vi "Sub Routing program.vi"(0 "queue Out in":refnum<queue>, 1 "FeedBack Channel":string[](array[string]), 2 "Load":refnum<vi>, 5 "reference in":refnum<vi>, 9 "Feature Step Enable":T1(array[cluster]), 11 "error in (no error)":errorcluster, 12 "Str Refnum":refnum<vi>, 14 "Pict Refnum":refnum<vi>) -> (3 "2D Picture":picture, 4 "Queue out":refnum<queue>, 6 "reference out":refnum<vi>, 10 "Result":bool, 15 "error out":errorcluster)   [LabVIEW 2015]
uses:
  Test  enqueue/AutoTest seq.ctl
  Galobal variable_TI.vi
  Project Setup/Globle Variable/GR_Servo.vi
panel:
  out "error out 2":errorcluster
  in  "Select Part":u16(ring) items=["CHECK BARCODE.jpg", "Difusser.jpg", "FIX BLACK PART.jpg", "FIXED PCB.jpg", "INSER KEYPAD.jpg", "IONIZE PCB.jpg", "light box ionization.jpg", "MOVE DOWN PART.jpg", "MOVING PART.jpg", "PART.jpg", "PUT PART ON FIXTURE.jpg"]
  out "Error Message":string
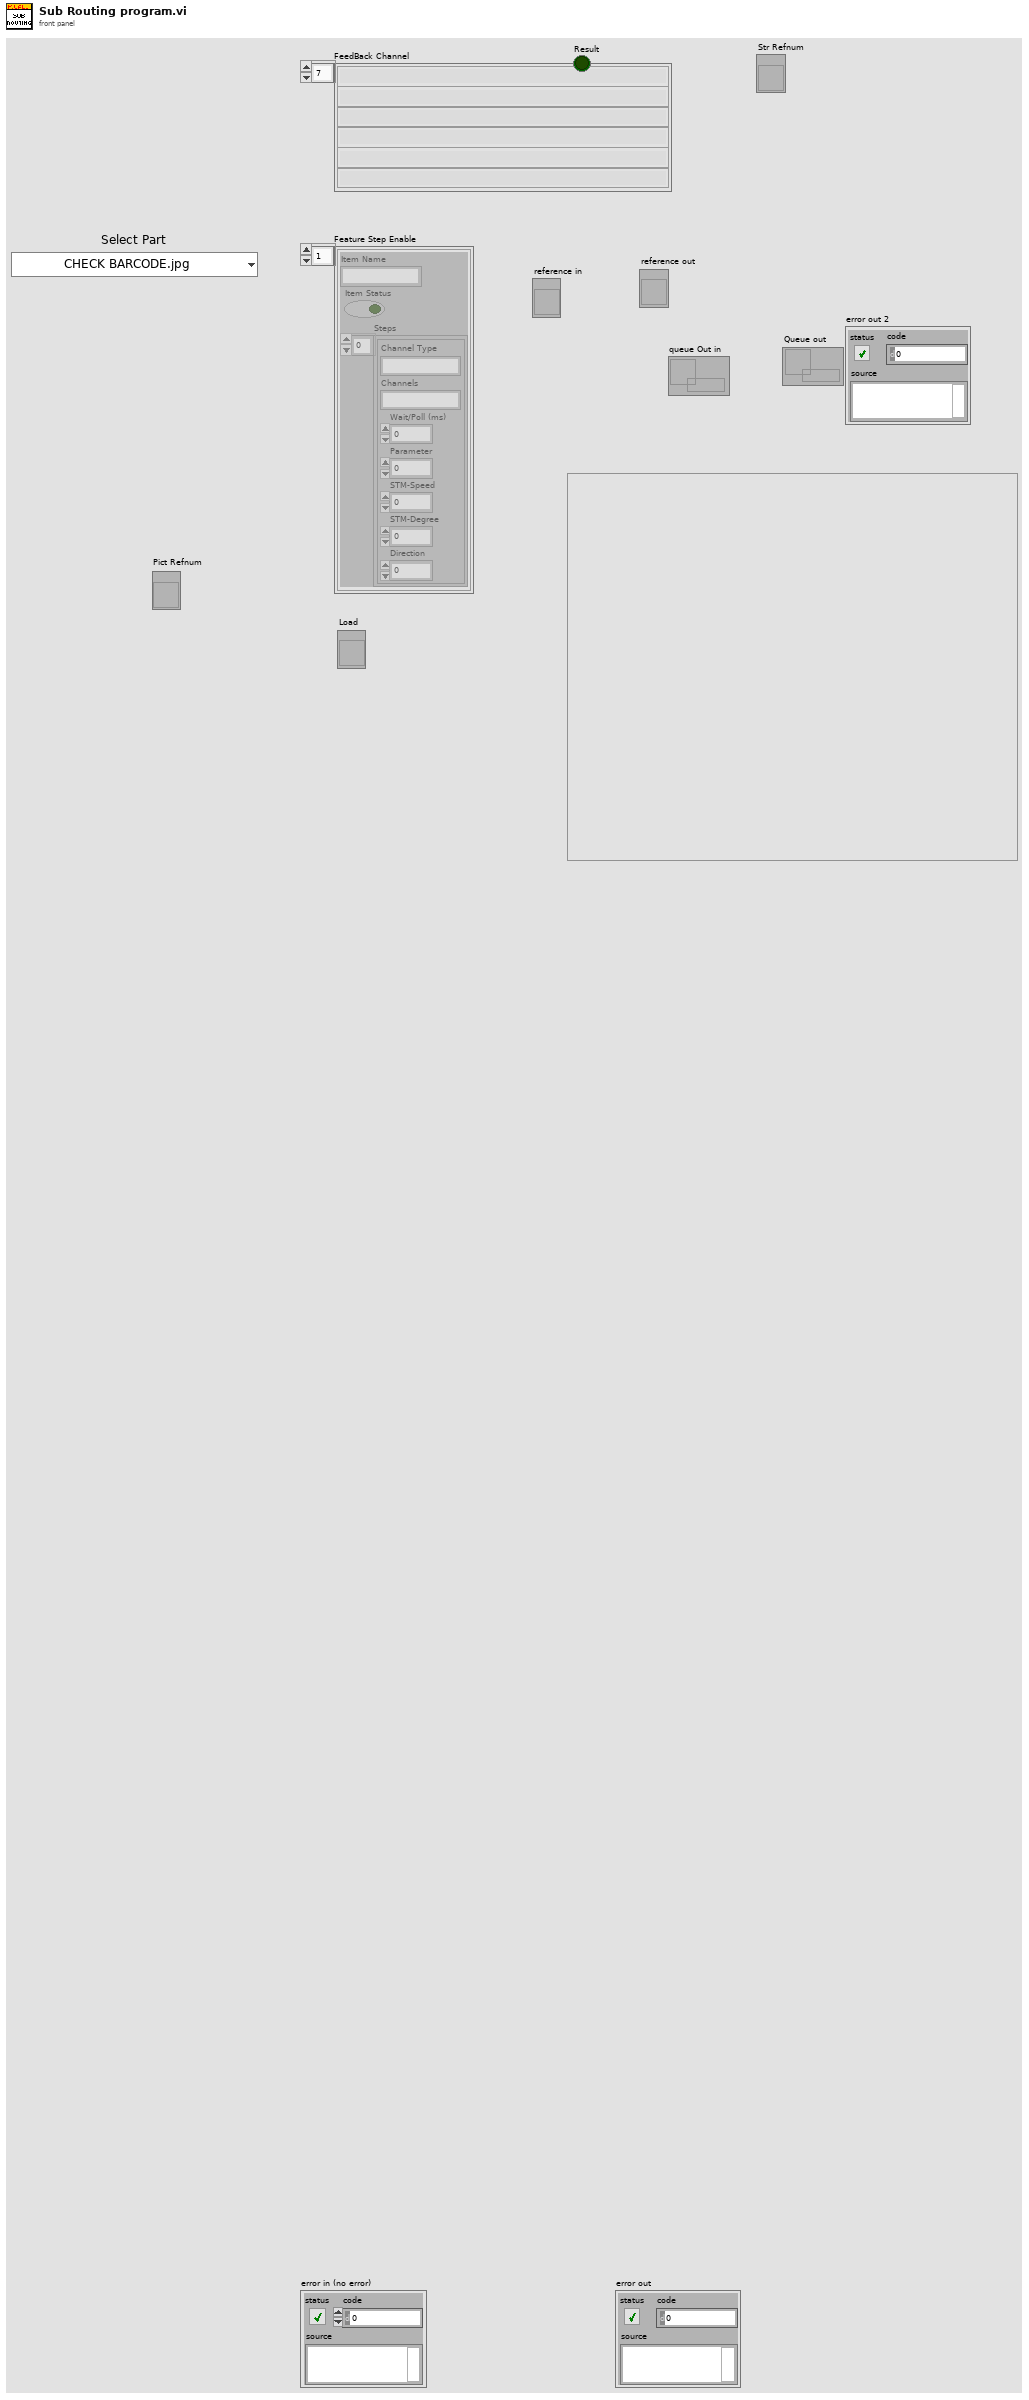
[diagram p1: front panel]
types:
  T1 = cluster{"Item Name":string, "Item Status":bool, "Steps":cluster{"Channel Type":string, "Channels":string, "Wait/Poll (ms)":u32, "Parameter":u8, "STM-Speed":i32, "STM-Degree":u32, "Direction":u8}[]}[]
  T2 = cluster{"Channel Type":string, "Channels":string, "Wait/Poll (ms)":u32, "Parameter":u8, "STM-Speed":i32, "STM-Degree":u32, "Direction":u8}[]
  T3 = cluster{"Start":bool, "Emergency ":bool, "Reset":bool, "Home":bool, "Safety":bool}
  T4 = typedef "LVPointTypeDef.ctl" = cluster{"Horizontal":i16, "Vertical":i16}
  T5 = typedef "LVBoundsTypeDef.ctl" = cluster{"Width":u32, "Height":u32}
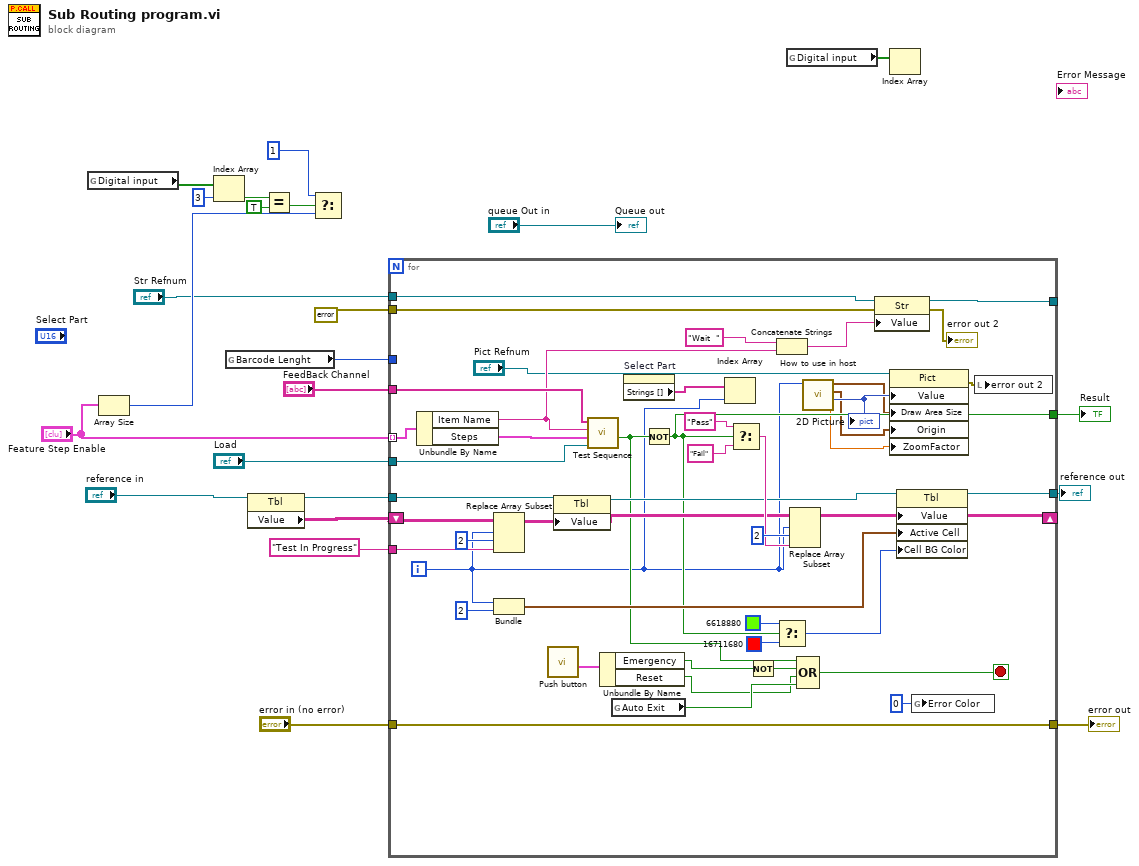
[diagram p0: block diagram]
diagram:
  n1 = global read "Galobal variable_TI.vi" "Digital input"() -> (w20:bool[])
  n2 = Array Size(array="Feature Step Enable") -> (size(s)=w5:i32)
  n3 = Index Array(array=w20, index=3) -> (element=w19:bool)
  n4 = global read "Galobal variable_TI.vi" "Barcode Lenght"() -> (w21:i32)
  n5 = property class="Tbl"(reference="reference in") -> (reference out=w9:refnum<vi>, "Value"=w12:string[][])  [unwired: 1 in, 1 out]
  n6 = Equal?(x=w19, y=TRUE) -> (x = y?=w16:bool)
  n7 = Select(t=1, s=w16, f=w5) -> ()  [unwired: 1 out]
  n8 = for {
    tunnel: "Feature Step Enable" -> [w69] mode=indexing
    tunnel: "FeedBack Channel" -> [w66]
    tunnel: w21 -> [_]
    shift-right: [w50] -> _
    shift-left: w12 -> [w62]
    tunnel: "Test In Progress" ("new element/subarray") -> [w61]
    tunnel: w9 -> [w60]
    tunnel: [w51] -> w8
    tunnel: "error in (no error)" -> [w49]
    tunnel: [w49] -> w6
    tunnel: [w44] -> w4
    tunnel: "Str Refnum" -> [w42]
    tunnel: [w41] -> _
    tunnel: errorcluster {"status"=FALSE, "code"=0, "source"=""} ("error in (no error)") -> [w35]
    tunnel: "Load" -> [w31]
    i -> [w30]
    stop <- w37 stop-if-true
    n9 = Unbundle By Name(w69) -> ("Item Name"=w39:string, "Steps"=w65:T2)
    n10 = Replace Array Subset(array=w62, new element=w61, index (row)=w30, index (col)=2 ("disabled index (col)")) -> (w57:string[][])
    n11 = Bundle(w30, 2) -> (w56:cluster{i32, i32})  [unwired: 1 in]
    n12 = call "Push button.vi"() -> ("Push Button"=w48:T3)  [unwired: 9 in, 2 out]
    n13 = property class="Tbl"(reference=w60, "Value"=w57) -> (reference out=w52:refnum<vi>)  [unwired: 1 in, 1 out]
    n14 = call "Test Sequence.vi"("FeedBack Channel"=w66, "Test Name"=w39, "Steps"=w65, "Load"=w31) -> ("Condition"=w45:bool)  [unwired: 3 in, 2 out]
    n15 = Unbundle By Name(w48) -> ("Emergency"=w47:bool, "Reset"=w28:bool)
    n16 = global read "Galobal variable_TI.vi" "Auto Exit"() -> (w29:bool)
    n17 = property on="Select Part" class="Ring (strict)"() -> ("Strings []"=w38:string[])  [unwired: 2 in, 2 out]
    n18 = Not(x=w45) -> (.not. x?=w44:bool)
    n19 = Index Array(array=w38, index=w30) -> ()  [unwired: 1 out]
    n20 = Select(t="Pass", s=w44, f="Fail") -> (s? t:f=w58:string)
    n21 = Not(x=w47) -> (.not. x?=w46:bool)
    n22 = Concatenate Strings("Wait  " ("string"), w39) -> (w40:string)
    n23 = Select(t=u32 6618880 ("Color Box"), s=w44, f=u32 16711680 ("Color Box")) -> (s? t:f=w53:u32)
    n24 = Replace Array Subset(array=w57, new element=w58, index (row)=w30, index (col)=2 ("disabled index (col)")) -> (w50:string[][])
    n25 = Compound Arithmetic op=OR(w45, w46, w28, w29) -> (w37:bool)
    n26 = call "How to use in host.vi"("Select Part"=w30) -> ("zoom"=w24:sgl, "2D Picture"=w34:picture, "output cluster"=w25:T4, "Draw Area Size"=w26:T5)  [unwired: 7 in]
    "2D Picture" <- w34
    n27 = property class="Str"(reference=w42, error in=w35, "Value"=w40) -> (reference out=w41:refnum<vi>, error out=→"error out 2":errorcluster)
    n28 = property class="Pict"(reference="Pict Refnum", "Value"=w34, "Draw Area Size"=w26, "Origin"=w25, "ZoomFactor"=w24) -> (error out=w32:errorcluster)  [unwired: 1 in, 1 out]
    n29 = property class="Tbl"(reference=w52, "Value"=w50, "Active Cell"=w56, "Cell BG Color"=w53) -> (reference out=w51:refnum<vi>)  [unwired: 1 in, 1 out]
    n30 = global write "GR_Servo.vi" "Error Color"(0 ("Error Color")) -> ()
    n31 = local write "error out 2"(w32) -> ()
  }
  "error out" <- w6
  "reference out" <- w8
  "Result" <- w4
  n32 = global read "Galobal variable_TI.vi" "Digital input"() -> (w22:bool[])
  n33 = Index Array(array=w22) -> ()  [unwired: 1 in, 1 out]
  "Queue out" <- "queue Out in"
